vi "massive settings for drivers vis.vi"() -> ()   [LabVIEW 2025]
doc: "This module set some VIs Properties programaticaly.\n\nVI Properties:\nGeneral\n Separate compiled code from source = TRUE\nExecution\n Allow debugging = FALSE\n Reentrancy = Non-reentrant execution\n Prefered Execution System = instrument I/O\n Enable automatic error handling = FALSE"
panel:
  in  "Disconnect VIs From Library?":bool
  in  "Folder VIs Path":path=path "C:/Users/Taboada.r248/Documents/LabVIEW Data/CHROMA-1905X-series-Driver/Files/Processed Files/Ready"
  # "YES"
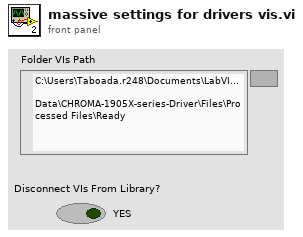
[diagram p1: front panel]
types:
  T1 = enum32{"Invalid", "Default", "Floating", "Floating/Auto-Hide", "Modal"}
  T2 = enum32{"invalid execution system", "user interface", "standard", "instrument i/o", "data acquisition", "other 1", "other 2", "same as caller"}
  T3 = enum32{"invalid lock state", "Not Locked", "Locked (No Password)", "Password-protected"}
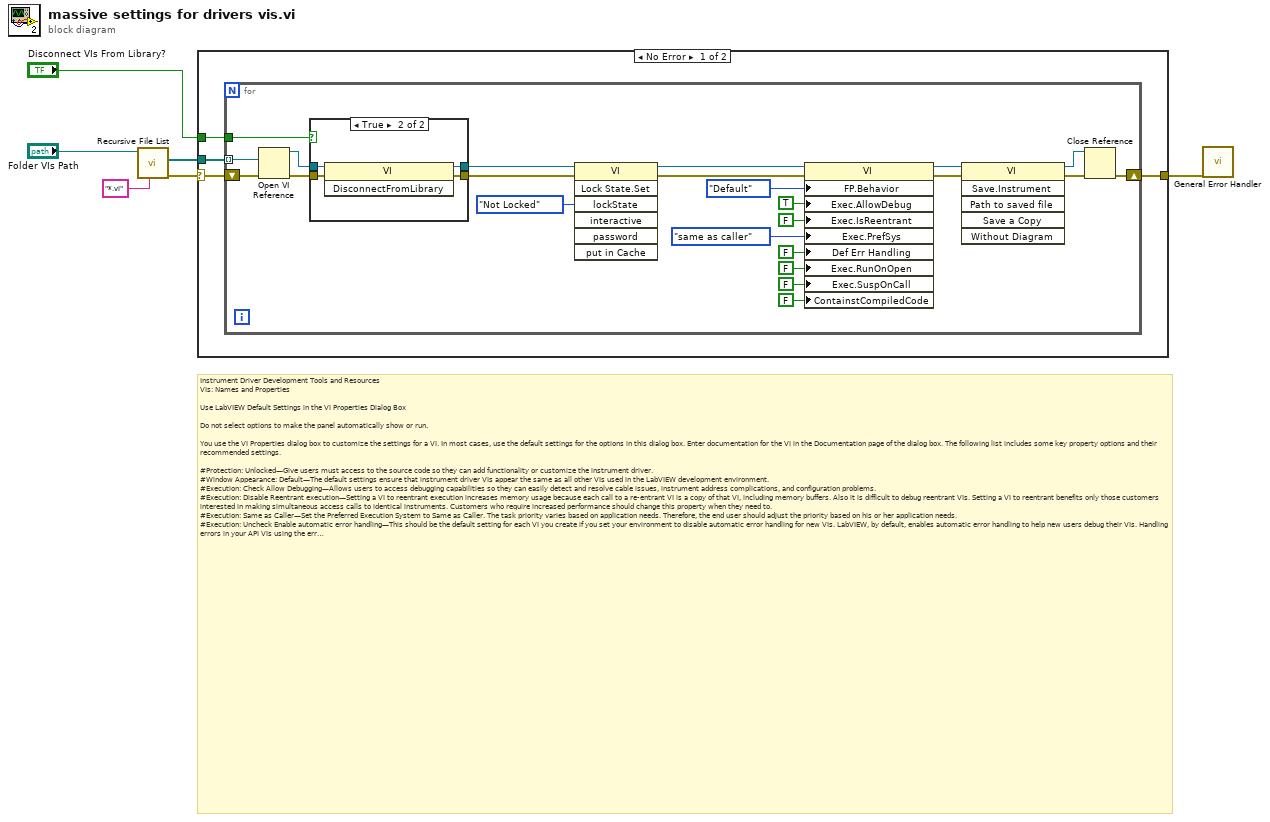
[diagram p0: block diagram]
diagram:
  # "Instrument Driver Development Tools and Resources \nVIs: Names and Properties\n \nUse LabVIEW Default Settings in the VI Properties Dialog Box\n\nDo not select options to make the panel automatically show or run.\n\nYou use the VI Properties dialog box to customize the settings for a VI. In most cases, use the default settings for the options in this dialog box. Enter documentation for the VI in the Documentation page of the dialog box. The following list includes some key property options and their recommended settings.\n\n#Protection: Unlocked—Give users must access to the source code so they can add functionality or customize the instrument driver.\n#Window Appearance: Default—The default settings ensure that instrument driver VIs appear the same as all other VIs used in the LabVIEW development environment.\n#Execution: Check Allow Debugging—Allows users to access debugging capabilities so they can easily detect and resolve cable issues, instrument address complications, and configuration problems.\n#Execution: Disable Reentrant execution—Setting a VI to reentrant execution increases memory usage because each call to a re-entrant VI is a copy of that VI, including memory buffers. Also it is difficult to debug reentrant VIs. Setting a VI to reentrant benefits only those customers interested in making simultaneous access calls to identical instruments. Customers who require increased performance should change this property when they need to.\n#Execution: Same as Caller—Set the Preferred Execution System to Same as Caller. The task priority varies based on application needs. Therefore, the end user should adjust the priority based on his or her application needs.\n#Execution: Uncheck Enable automatic error handling—This should be the default setting for each VI you create if you set your environment to disable automatic error handling for new VIs. LabVIEW, by default, enables automatic error handling to help new users debug their VIs. Handling errors in your API VIs using the error in and error out cluster parameters ensures errors are properly reported to users.\n#Execution: Uncheck Run when Opened—When used interactively, users should control when the VI runs.\n#Execution: Uncheck Suspend when Called—Instrument Driver VIs never should be suspended when called.\n\nSource: https://www.ni.com/en/support/downloads/instrument-drivers/tools-resources/instrument-driver-guidelines/vis-names-and-properties.html"
  n1 = call <vilib>:"Recursive File List.vi"("pattern"="*.vi", "Folder Path"="Folder VIs Path") -> ("error out"=w1:errorcluster, "All Files in Dir"=w5:path[])  [unwired: 5 in, 3 out]
  n2 = case shown="No Error" w1 {
    selector: w1 -> [w7 w40]
    tunnel: w5 -> [w10 _]
    tunnel: [w9 w40] -> w4
    tunnel: "Disconnect VIs From Library?" -> [w8 _]
    frame No Error {
      n3 = for {
        tunnel: w10 -> [w33] mode=indexing
        shift-right: [w31] -> w9
        shift-left: w7 -> [w32]
        tunnel: w8 -> [w11]
        n4 = Open VI Reference(vi path=w33, error in (no error)=w32) -> (vi reference=w14:refnum<vi>, error out=w15:errorcluster)  [unwired: 4 in]
        n5 = case shown="True" w11 {
          tunnel: w15 -> [w35 w39]
          tunnel: w14 -> [w34 w38]
          tunnel: [w34 w37] -> w13
          tunnel: [w35 w36] -> w12
          frame False {
          }
          frame True {
            n6 = invoke class="VI" method="DisconnectFromLibrary"(reference=w38, error in=w39) -> (reference out=w37:refnum<vi>, error out=w36:errorcluster)  [unwired: 1 in, 1 out]
          }
        }
        n7 = invoke class="VI" method="Lock State.Set"(reference=w13, error in=w12, "lockState"=T3."Not Locked" ("Lock State")) -> (reference out=w24:refnum<vi>, error out=w18:errorcluster)  [unwired: 4 in, 5 out]
        n8 = property class="VI"(reference=w24, error in=w18, "FP.Behavior"=T1."Default" ("Front Panel Window:Behavior"), "Exec.AllowDebug"=TRUE ("Execution:Allow Debugging"), "Exec.IsReentrant"=FALSE ("Execution:Is Reentrant"), "Exec.PrefSys"=T2."same as caller" ("Execution:Preferred Exec System"), "Def Err Handling"=FALSE ("Automatic Error Handling"), "Exec.RunOnOpen"=FALSE ("Execution:Is Reentrant"), "Exec.SuspOnCall"=FALSE ("Execution:Suspend On Call"), "ContainstCompiledCode"=FALSE ("Contains Compiled Code")) -> (reference out=w17:refnum<vi>, error out=w16:errorcluster)
        n9 = invoke class="VI" method="Save.Instrument"(reference=w17, error in=w16) -> (reference out=w29:refnum<vi>, error out=w30:errorcluster)  [unwired: 4 in, 4 out]
        n10 = Close Reference(reference=w29, error in (no error)=w30) -> (error out=w31:errorcluster)
      }
    }
    frame Error {
    }
  }
  n11 = call <vilib>:"General Error Handler.vi"("error in (no error)"=w4) -> ()  [unwired: 10 in, 5 out]
